vi "Read Type.vi"(8 "error in":errorcluster, 11 "channel in":refnum<class "Channel.lvclass">) -> (0 "error out":errorcluster, 2 "type":T1, 3 "channel out":refnum<class "Channel.lvclass">)   [LabVIEW 2020, in "Scan Engine Scripting.lvlib" / "Channel.lvclass"]
uses:
  Channel.lvclass
  Type.ctl
  Channel.lvclass/Channel.ctl
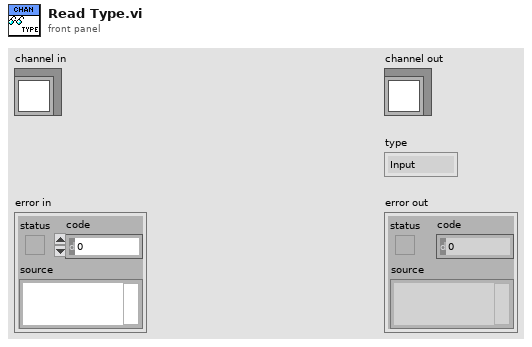
[diagram p1: front panel]
types:
  T1 = typedef "Scan Engine Scripting.lvlib/Channel.lvclass/Type.ctl" = enum16{"Input", "Output"}
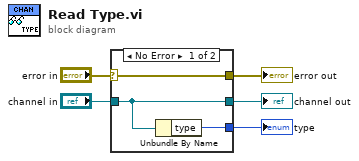
[diagram p0: block diagram]
diagram:
  n1 = case shown="No Error" "error in" {
    selector: "error in" -> [w8 w9]
    tunnel: [w8 w9] -> w4
    tunnel: [w7 w10] -> w2
    tunnel: "channel in" -> [w7 w10]
    tunnel: [w6 _] -> w1
    frame No Error {
      n2 = Unbundle By Name(w7) -> ("type"=w6:T1)
    }
    frame Error {
    }
  }
  "error out" <- w4
  "channel out" <- w2
  "type" <- w1
